vi "Close.vi"(8 "error in (no error)":errorcluster, 11 "Generic Data Acquisition in":refnum<class "Generic Data Acquisition.lvclass">) -> (0 "error out":errorcluster, 3 "Generic Data Acquisition out":refnum<class "Generic Data Acquisition.lvclass">)   [LabVIEW 2016, in "Generic Data Acquisition.lvlib" / "Generic Data Acquisition.lvclass"]
uses:
  Generic Data Acquisition.lvclass
  Abstract Sensor/Abstract Sensor.lvclass
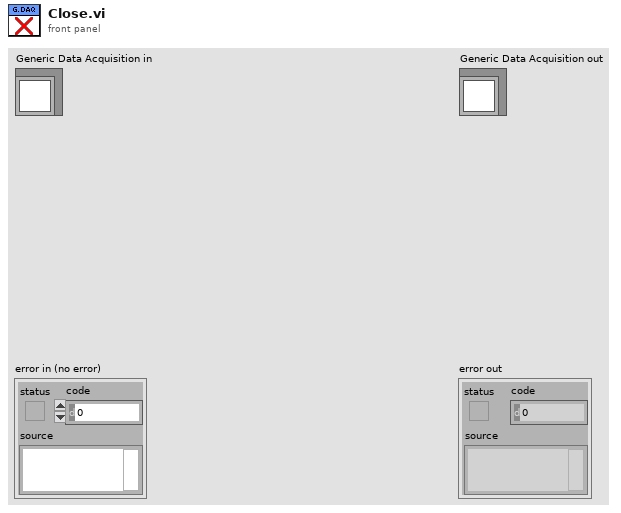
[diagram p1: front panel]
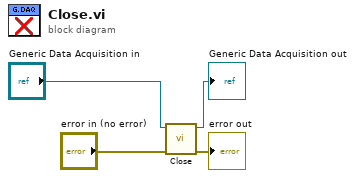
[diagram p0: block diagram]
diagram:
  n1 = call-parent "Close.vi"("error in (no error)"="error in (no error)", "Abstract Sensor in"="Generic Data Acquisition in") -> ("error out"=→"error out":errorcluster, "Abstract Sensor out"=→"Generic Data Acquisition out":refnum<class "Generic Data Acquisition.lvclass">)  [unwired: 8 in]
